vi "HTVacuumGUI.CalcColor.vi"(1 "Input-Value":i32, 3 "Color1":u32, 8 "Color2":u32, 9 "Color3":u32) -> (15 "Output-Value":u32)   [LabVIEW 2014, in "HTVacuumGUI.lvlib"]
uses:
  HTVacuumGUI.lvlib
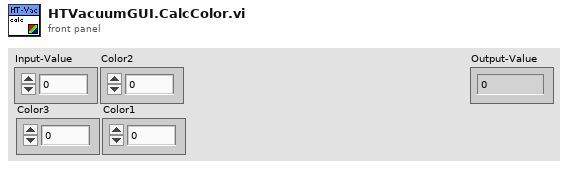
[diagram p1: front panel]
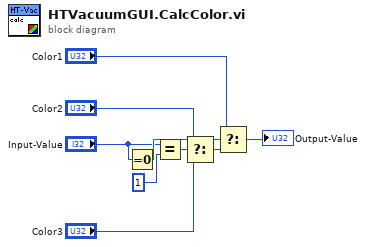
[diagram p0: block diagram]
diagram:
  n1 = Equal To 0?(x="Input-Value") -> (x = 0?=w6:bool)
  n2 = Equal?(x="Input-Value", y=u32 1) -> (x = y?=w8:bool)
  n3 = Select(t="Color2", s=w8, f="Color3") -> (s? t:f=w9:u32)
  n4 = Select(t="Color1", s=w6, f=w9) -> (s? t:f=→"Output-Value":u32)
